vi "configureOutput.vi"(6 "sofwareTrigger?":bool, 8 "error in (no error)":errorcluster, 9 "Data":variant, 10 "Config":T1, 11 "DDSOutput in":refnum<class "DDSOutput.lvclass">) -> (0 "error out":errorcluster, 3 "DDSOutput out":refnum<class "DDSOutput.lvclass">)   [LabVIEW 2011, in "Hardware.lvlib" / "Channels.lvlib" / "DDSOutput.lvclass"]
doc: "Data is an array of varient clusters. One varient cluster per channel.\n\nVariant is a 2D array { {Time, Freq, Amplitude,Phase},...}"
uses:
  DDSOutput.lvclass
  DDSOutput.lvclass/DDSOutput.ctl
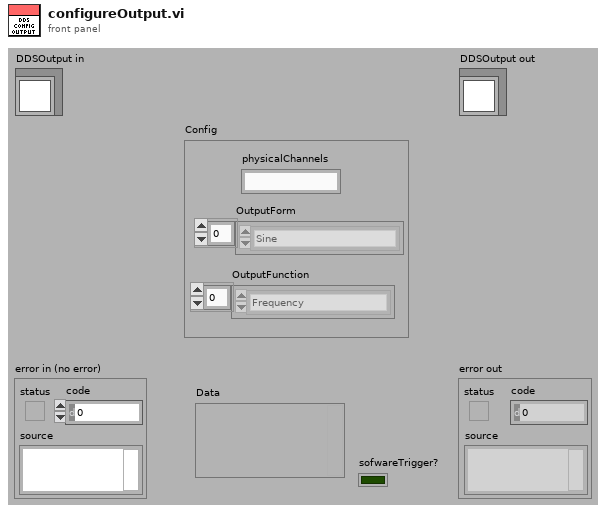
[diagram p1: front panel]
types:
  T1 = cluster{"OutputForm":enum16{"Sine", "Square", "Triangle", "Arbitrary"}[], "OutputFunction":enum16{"Frequency", "Ramp", "Sequence"}[], "physicalChannels":string}
  T2 = enum16{"Sine", "Square", "Triangle", "Arbitrary"}[]
  T3 = cluster{"OutputForm":enum16{"Sine", "Square", "Triangle", "Arbitrary"}[], "OutputFunction":enum16{"Frequency", "Ramp", "Sequence"}[], "physicalChannels":string[]}
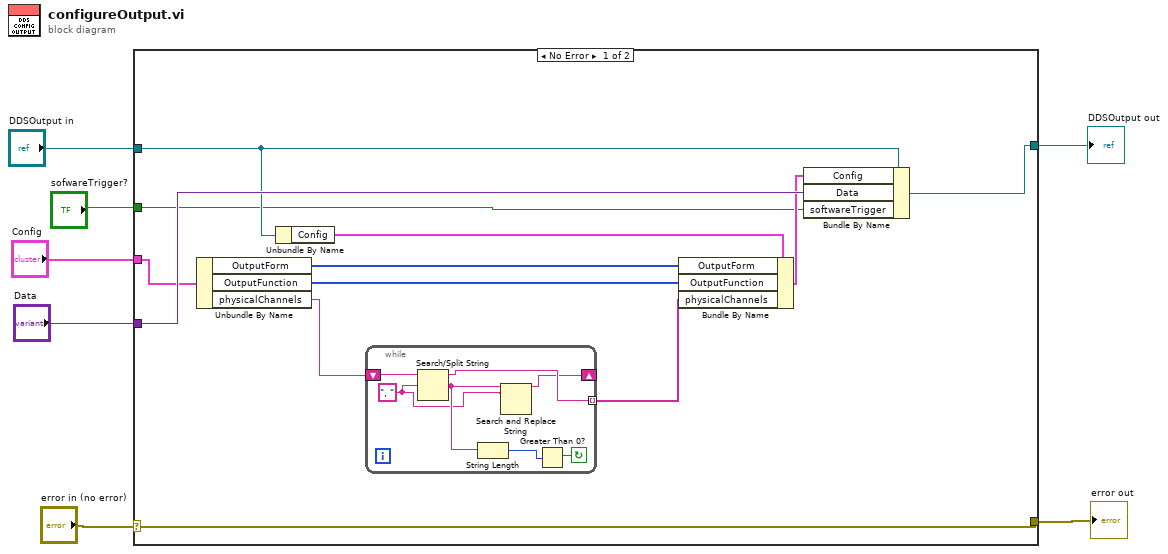
[diagram p0: block diagram]
diagram:
  n1 = case shown="No Error" "error in (no error)" {
    selector: "error in (no error)" -> [w17 w28]
    tunnel: [w17 w28] -> w6
    tunnel: [w19 w27] -> w4
    tunnel: "DDSOutput in" -> [w14 w27]
    tunnel: "Data" -> [w18 _]
    tunnel: "Config" -> [w15 _]
    tunnel: "sofwareTrigger?" -> [w8 _]
    frame No Error {
      n2 = Unbundle By Name(w15) -> ("OutputForm"=w11:T2, "OutputFunction"=w10:enum16{"Frequency", "Ramp", "Sequence"}[], "physicalChannels"=w16:string)
      n3 = Unbundle By Name(w14) -> ("Config"=w13:T3)
      n4 = while {
        shift-right: [w22] -> _
        shift-left: w16 -> [w26]
        tunnel: [w25] -> w12 mode=indexing
        stop <- w20 continue-if-true
        w23 = ", "
        n5 = Search/Split String(string=w26, search string/char (-)=w23) -> (substring before match=w25:string, match + rest of string=w24:string)  [unwired: 1 in, 1 out]
        n6 = String Length(string=w24) -> (length=w21:i32)
        n7 = Search and Replace String(input string=w24, search string=w23) -> (result string=w22:string)  [unwired: 6 in, 3 out]
        n8 = Greater Than 0?(x=w21) -> (x > 0?=w20:bool)
      }
      n9 = Bundle By Name(cluster=w13, "OutputForm"=w11, "OutputFunction"=w10, "physicalChannels"=w12) -> (w9:T3)
      n10 = Bundle By Name(cluster=w14, "Config"=w9, "Data"=w18, "softwareTrigger"=w8) -> (w19:refnum<class "DDSOutput.lvclass">)
    }
    frame Error {
    }
  }
  "error out" <- w6
  "DDSOutput out" <- w4
